vi "Pup_upper.vi"(9 "K11":fxp<+,32,16>, 10 "output valid 12":bool, 11 "E11":fxp<+,32,16>) -> (2 "output valid 11":bool, 3 "Pup11":fxp<+,32,16>)   [LabVIEW 2020]
uses:
  <vilib>/rvi/FXPMathLib/FxpSub/XNode/nifxpmath_Sub.xnode
  <vilib>/rvi/FXPMathLib/FxpMul/XNode/nifxpmath_Multiplier.xnode
  <vilib>/rvi/FXPMathLib/sim/FxpSim.dll
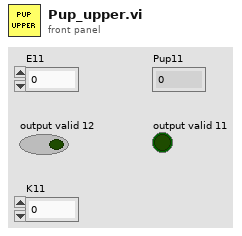
[diagram p1: front panel]
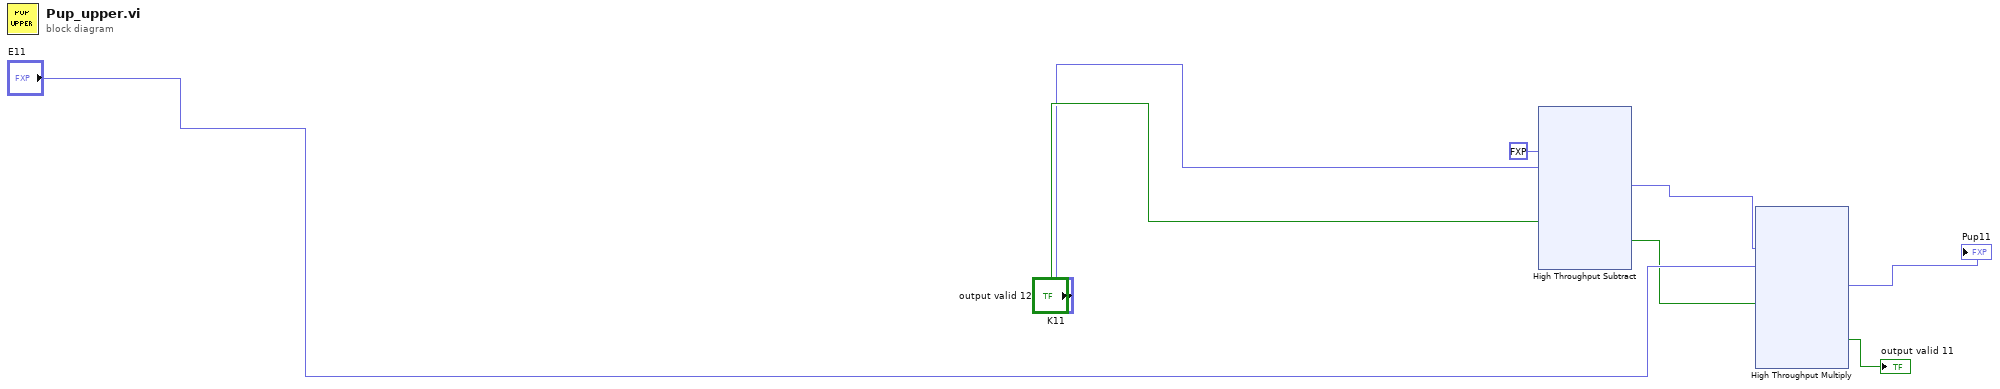
[diagram p0: block diagram]
diagram:
  n1 = xnode "High Throughput Subtract"("x"=fxp<+,8,8> 1.0, "y"="K11", "input valid"="output valid 12") -> ("x-y"=w4:fxp<+/-,32,16>, "output valid"=w6:bool)  [unwired: 1 in, 1 out]
  n2 = xnode "High Throughput Multiply"("x"=w4, "y"="E11", "input valid"=w6) -> ("x*y"=→"Pup11":fxp<+,32,16>, "output valid"=→"output valid 11":bool)  [unwired: 1 in, 1 out]
